vi "test.vi"() -> ()   [LabVIEW 2018]
uses:
  tcpServer.lvclass
  tcpServer.lvclass/tcpServer.ctl
panel:
  in  "stop":bool
  in  "serverPort 3":u16=10
  out "serverPort 2":u16
  out "serverPort":u16
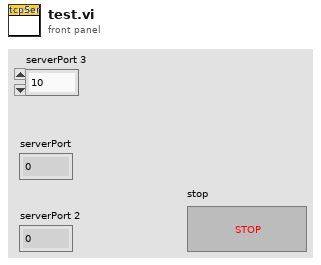
[diagram p1: front panel]
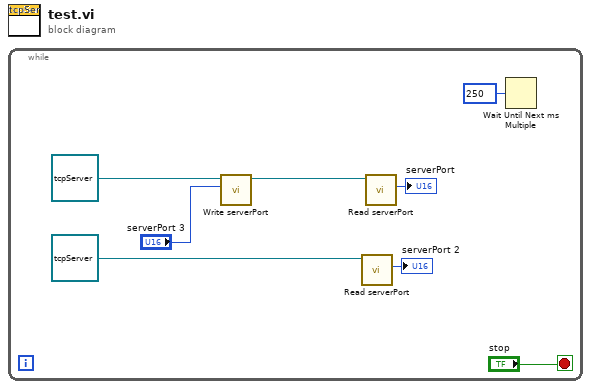
[diagram p0: block diagram]
diagram:
  n1 = while {
    stop <- "stop" stop-if-true
    n2 = call "Write serverPort.vi"("serverPort"="serverPort 3", "tcpServer in"=refnum<class "tcpServer.lvclass"> refnum ("tcpServer.lvclass")) -> ("tcpServer out"=w7:refnum<class "tcpServer.lvclass">)  [unwired: 8 in, 1 out]
    n3 = call "Read serverPort.vi"("tcpServer in"=refnum<class "tcpServer.lvclass"> refnum ("tcpServer.lvclass")) -> ("serverPort"=→"serverPort 2":u16)  [unwired: 8 in, 2 out]
    n4 = call "Read serverPort.vi"("tcpServer in"=w7) -> ("serverPort"=→"serverPort":u16)  [unwired: 8 in, 2 out]
    n5 = Wait Until Next ms Multiple(millisecond multiple=u32 250) -> ()  [unwired: 1 out]
  }
